vi "MTS_Main.vi"() -> ()   [LabVIEW 8.6]
panel:
  out "Pattern Y":dbl[](array[numeric])
  out "Pattern X":dbl[](array[numeric])
  out "Active pt3":path
  in  "Axis":enum32{"x-y", "x-z", "y-z"}(ring)
  in  "Save Files":bool=TRUE
  out "Intensity (a.u.)":dbl=1.0 format="%.02f"
  out "Detector2":bool
  out "Detector1":bool
  out "Excitation":bool
  in  "Measurement Time (ms)":i32=10
  in  "Open MSW":bool
  in  "New MSW":bool
  out "Workspace":path
  in  "WS File Tree":string(tree)
  out "Stop Measurement":bool
  in  "Learning loop":bool=TRUE
  in  "ShowTab":T1(tab)=enum."Auto Measurement"
  out "Video":u8[][](graph)
  in  "Find Mols":bool
  out "Image":i32[][](graph)
  in  "Save Color Image":bool
  out "AM image":T2(plugin-control)
  out "Histogram":i32[][](graph)
  out "Trace":i32[][](graph)
  out "FiFo Overrun":bool
  in  "SCANNER EMERGENCY":bool
  out "Measure. time [s]":i32
  in  "Scanner Divider":i32=2
  out "y":dbl format="%.1f nm"
  out "x":dbl format="%.1f nm"
  in  "x-Pixel":u16=100
  in  "y-Pixel":u16=100
  in  "Picture size":dbl=50.0 format="%1.1f um"
  in  "Picture size 2":dbl=50.0 format="%1.1f um"
  in  "Z-Position":dbl=50.0 caption="Z" format="%1.3f um"
  in  "Y-Position":dbl=50.0 caption="Y" format="%1.3f um"
  in  "X-Position":dbl=50.0 caption="X" format="%1.3f um"
  out "Do Measurement":T3(ring)
  in  "Point Measurement":bool
  in  "Aquire Image":bool
  in  "Settings":bool
  in  "PI E710 Port":u16(ring) items=["COM1", "COM2", "COM3", "COM4", "COM5", "COM6", "COM7", "COM8", "COM9"]
  in  "Move Stage":bool
  out "MeasRunig":bool
  in  "Stop Program":bool
  out "Global Stop":bool
  # "Workspace"
  # "Shutter:"
  # "Image Scan Settings"
  # "Point Measurement Settings"
  # "upper left corner/ Point Position"
  # "Pixelsize"
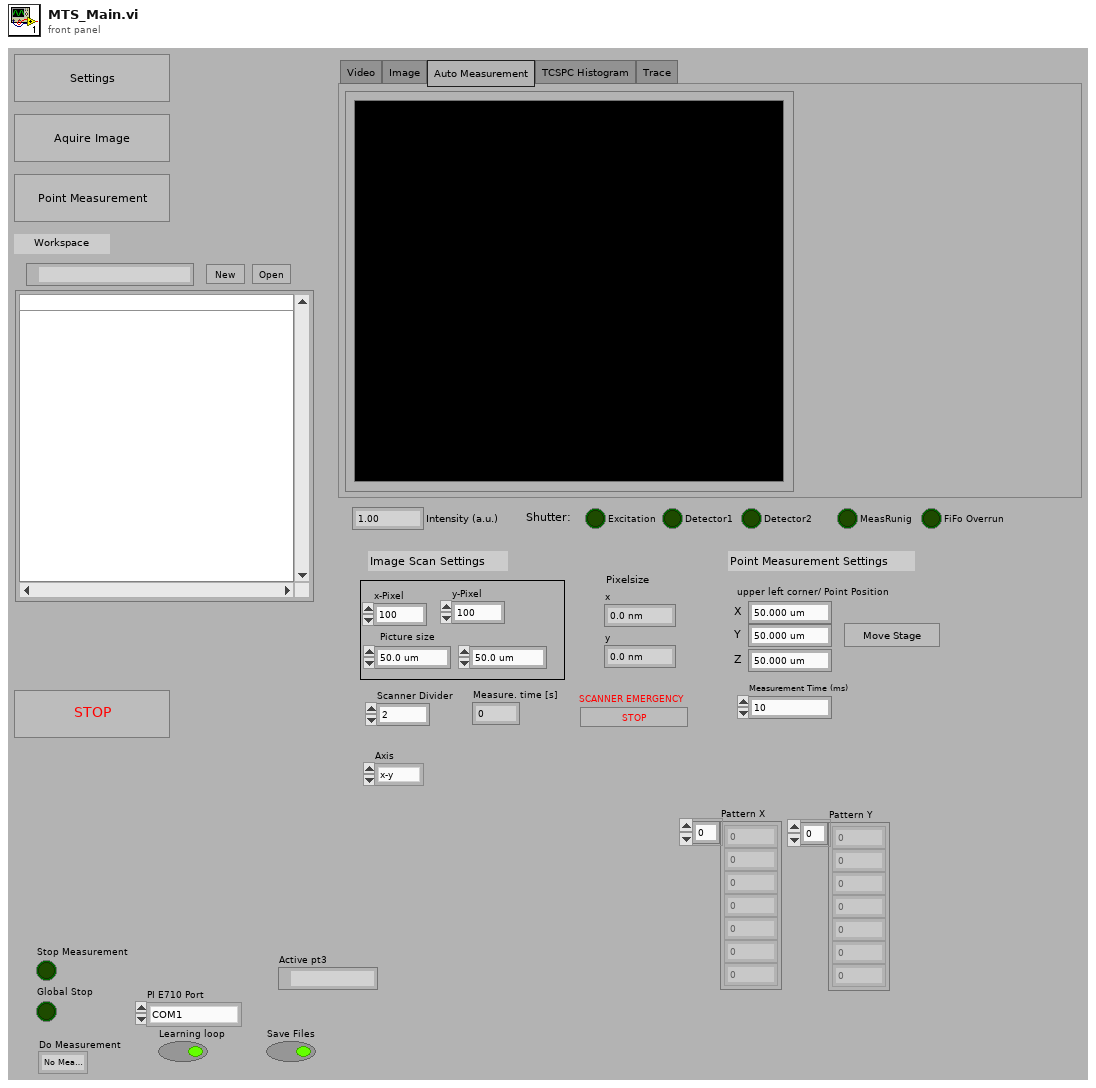
[diagram p1: front panel]
types:
  T1 = enum32{"Video", "Image", "Auto Measurement", "TCSPC Histogram", "Trace"}
  T2 = typedef "IMAQ Image.ctl" = refnum<image>
  T3 = enum16{"No Measurement", "Aquire Image", "Point Measurement", "Multi Measurement", "Save Color Image", "Find Single Mol."}
  T4 = enum16{"CAN_Baud_1M", "CAN_BAUD_500K", "CAN_BAUD_250K", "CAN_BAUD_125K", "CAN_BAUD_100K", "CAN_BAUD_50K", "CAN_BAUD_20K", "CAN_BAUD_10K", "CAN_BAUD_5K", "User"}
  T5 = enum16{"No Measurement", "Aquire Image", "Point Measurement", "Multi Measurement"}
  T6 = typedef "Image Type" = u32
  T7 = cluster{"Height":u32, "Width":u32, "Pixel Depth":u32}
  T8 = cluster{"Dev":i32, "SerNo":string, "HW_Model":string, "HW_Version":string}[]
  T9 = enum32{"Video", "Image", "TCSPC Histogram", "Trace"}
  T10 = cluster{"ID":u32, "MSG type":enum8{"STD, NO RTR", "STD,RTR", "XTD, NO RTR", "XTD, RTR"}, "LEN":u8, "DATA":u8[]}
  T11 = enum16{"No Measurement", "Aquire Image", "Point Measurement", "Multi Measurement", "Save Color Image"}
  T12 = enum16{"Get (Default)", "Set Workspace", "Append File", "Change Comment"}
  T13 = enum16{"unknown", "pt3 File", "png Image", "bmp Image"}
  T14 = cluster{"File No":i32, "File Path":path, "Parent File":i32, "File Type":enum16{"unknown", "pt3 File", "png Image", "bmp Image"}, "Measurement Type":enum16{"not a pt3 File", "Image File", "Point Measurement", "Auto Point"}, "Upper Left":cluster{"x-Position":dbl, "y-Position":dbl, "z-Position":dbl}, "Pixels":i32[], "Picture Size":dbl[], "Scan Axis":enum32{"x-y", "x-z", "y-z"}}[]
  T15 = typedef "LVPoint32TypeDef.ctl" = cluster{"Horizontal":i32, "Vertical":i32}
  T16 = cluster{"Shift":bool, "Ctrl":bool, "Alt":bool, "Cmd":bool, "Opt":bool}
  T17 = cluster{"File No":i32, "File Path":path, "Parent File":i32, "File Type":enum16{"unknown", "pt3 File", "png Image", "bmp Image"}, "Measurement Type":enum16{"not a pt3 File", "Image File", "Point Measurement", "Auto Point"}, "Upper Left":cluster{"x-Position":dbl, "y-Position":dbl, "z-Position":dbl}, "Pixels":i32[], "Picture Size":dbl[], "Scan Axis":enum32{"x-y", "x-z", "y-z"}}
  T18 = enum16{"not a pt3 File", "Image File", "Point Measurement", "Auto Point"}
  T19 = cluster{"x-Position":dbl, "y-Position":dbl, "z-Position":dbl}
  T20 = cluster{"X-Position":dbl, "Y-Position":dbl, "Z-Position":dbl}
  T21 = cluster{"Picture Size":dbl[], "Pixels":i32[], "Upper Left":cluster{"x-Position":dbl, "y-Position":dbl, "z-Position":dbl}}
  T22 = cluster{"Dev":i32, "SerNo":string, "HW_Model":string, "HW_Version":string}
  T23 = cluster{"Comment":string, "RangeNo":i32, "Offset":i32, "AcquisitionTime (ms)":i32, "HardwareSerial":i32, "SyncDivider":i32, "Resolution (ns)":sgl, "CFD Settings":cluster{"Ch0 Level":i32, "Ch0 ZeroX":i32, "Ch1 Level":i32, "Ch1 ZeroX":i32}, "InpRate0":i32, "InpRate1":i32}
  T24 = cluster{"X-Position":dbl, "Z-Position":dbl, "Y-Position":dbl}
  T25 = cluster{"Ident":string, "Format Version":string, "Creator Name":string, "Creator Version":string, "File Time":string, "Comment":string, "RangeNo":i32, "Offset":i32, "AcquisitionTime (ms)":i32, "HardwareSerial":i32, "SyncDivider":i32, "Resolution (ns)":sgl, "CFD Settings":cluster{"Ch0 Level":i32, "Ch0 ZeroX":i32, "Ch1 Level":i32, "Ch1 ZeroX":i32}, "InpRate0":i32, "InpRate1":i32}
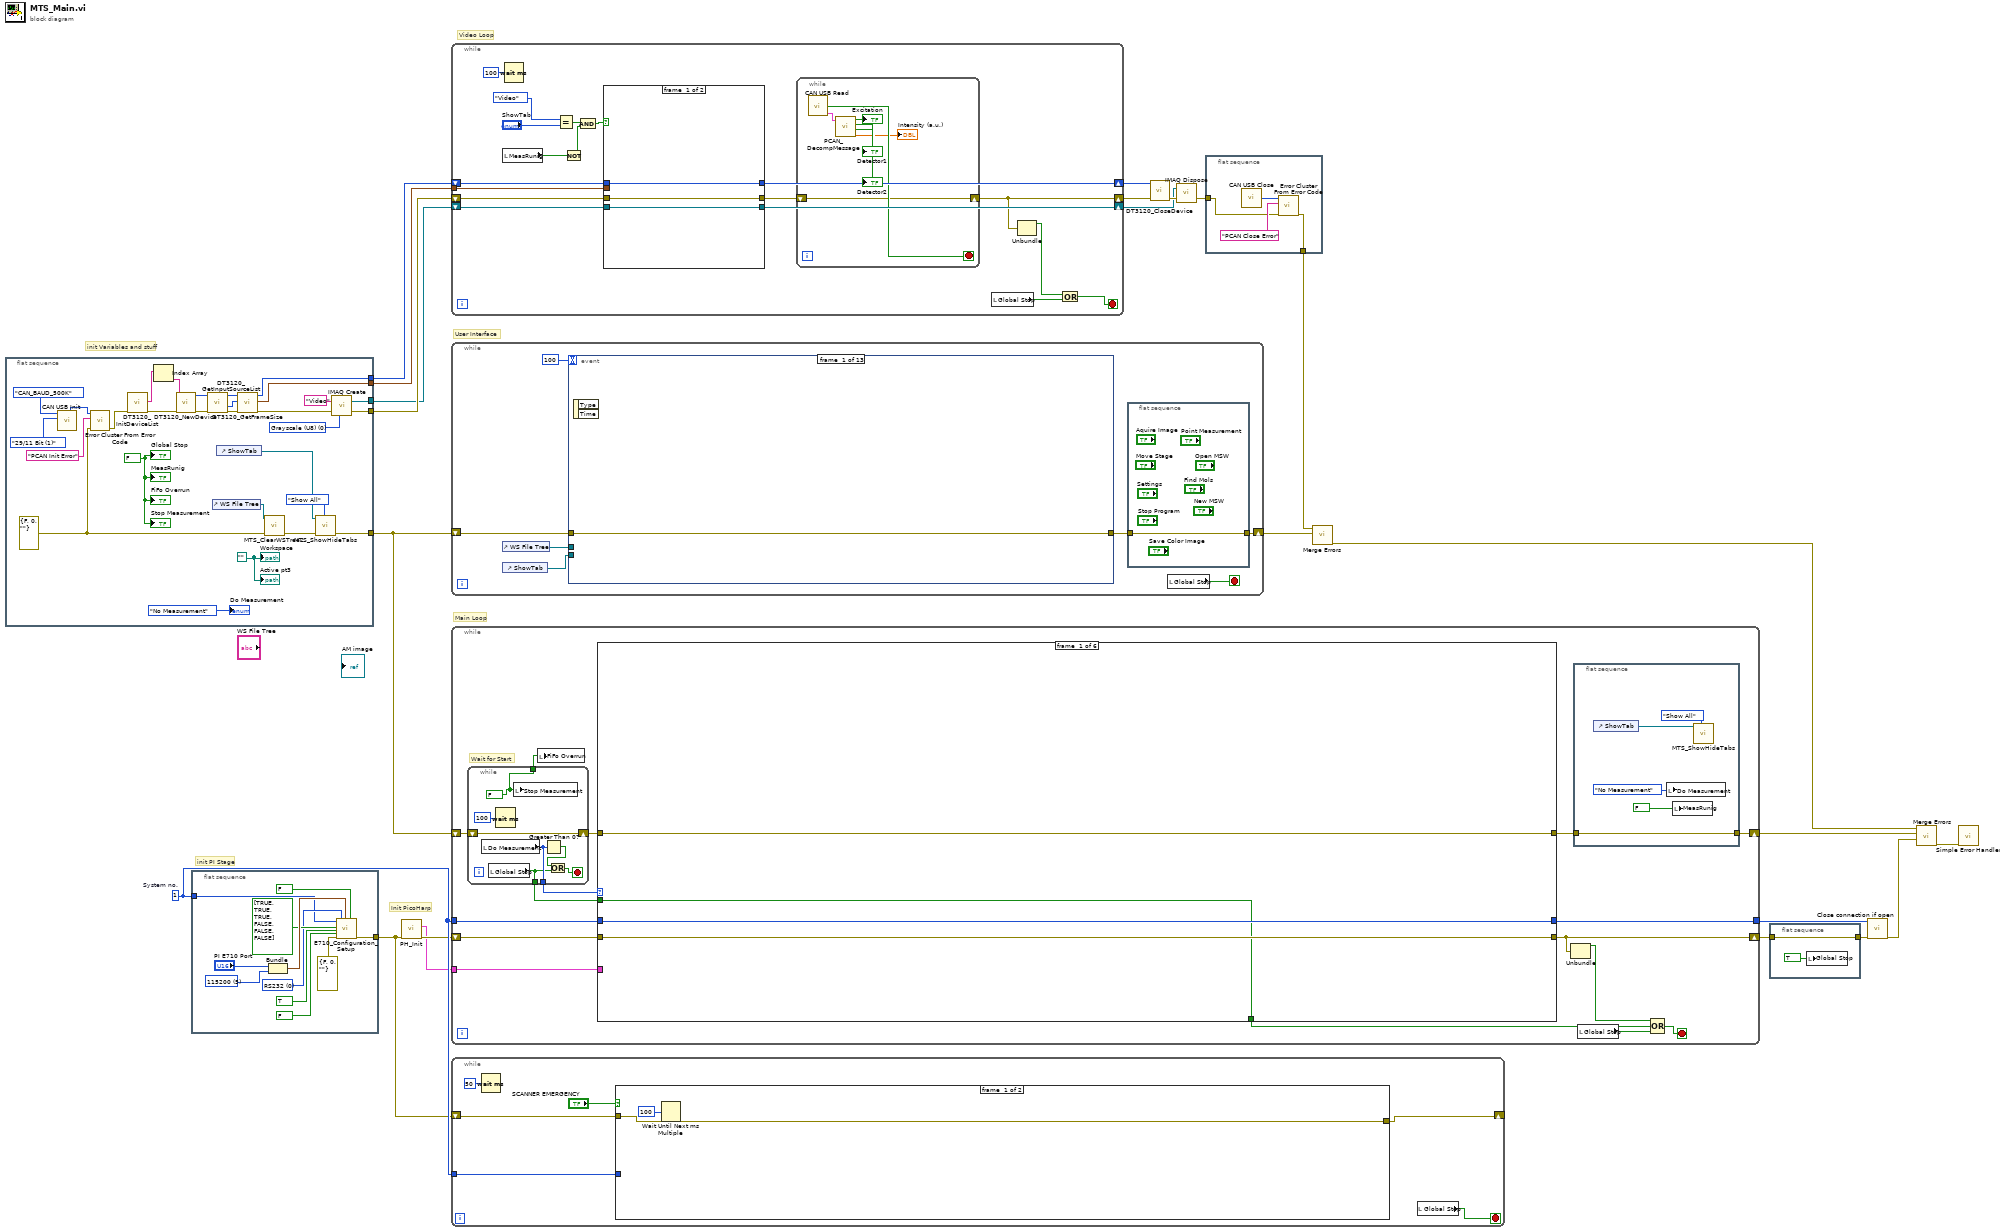
[diagram p0: block diagram]
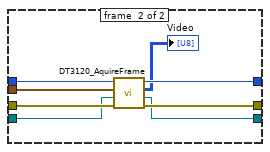
[diagram p2: hidden frame]
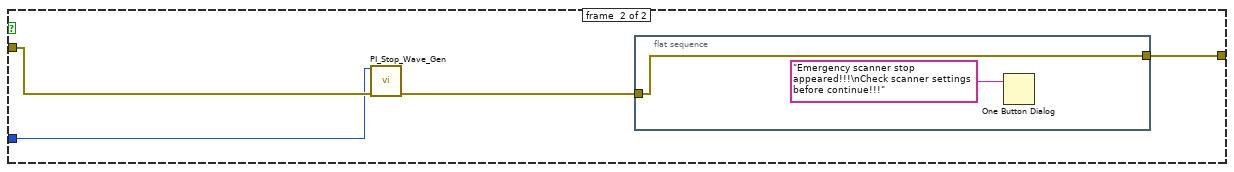
[diagram p3: hidden frame]
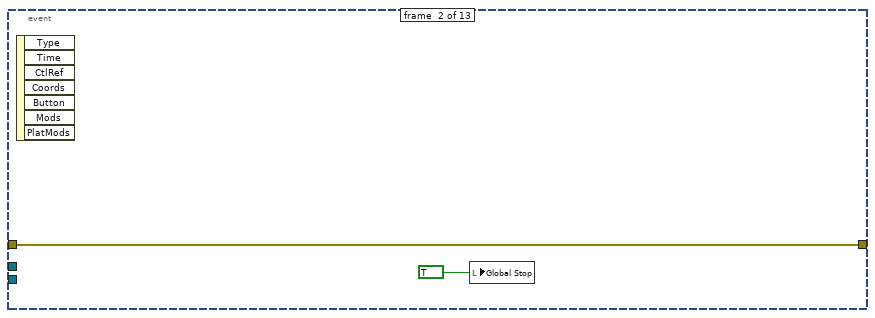
[diagram p4: hidden frame]
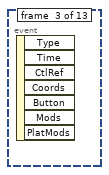
[diagram p5: hidden frame]
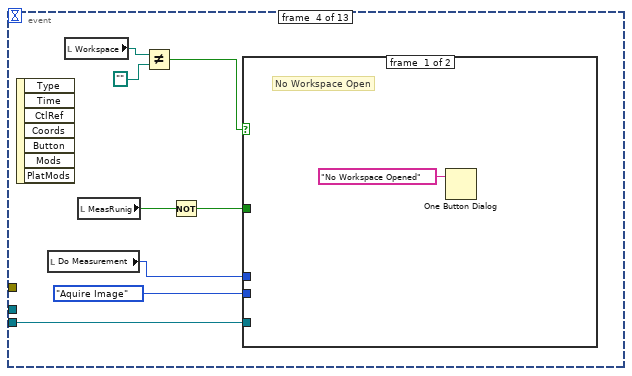
[diagram p6: hidden frame]
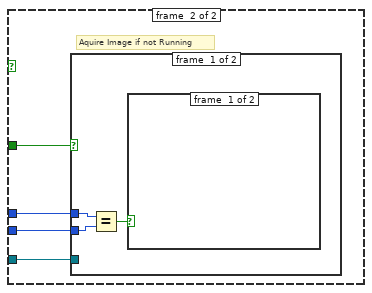
[diagram p7: hidden frame]
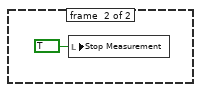
[diagram p8: hidden frame]
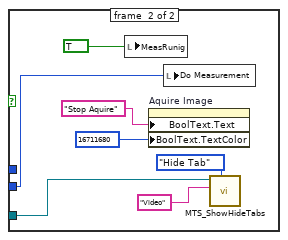
[diagram p9: hidden frame]
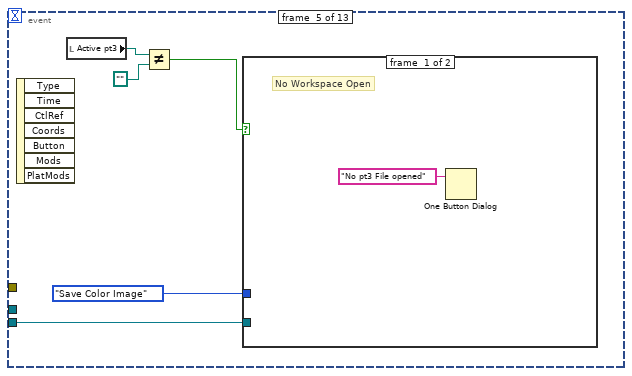
[diagram p10: hidden frame]
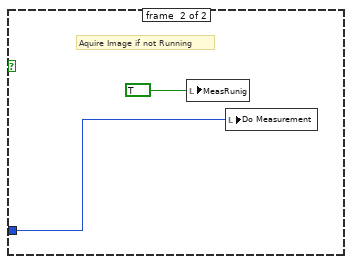
[diagram p11: hidden frame]
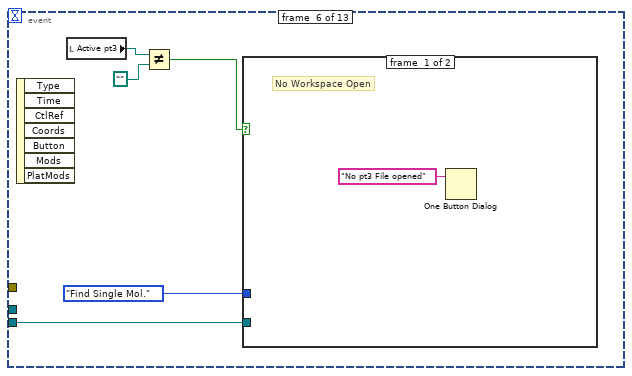
[diagram p12: hidden frame]
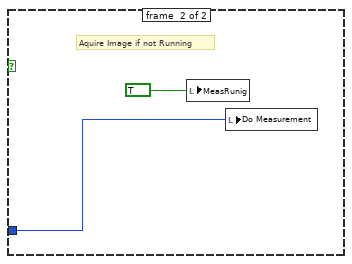
[diagram p13: hidden frame]
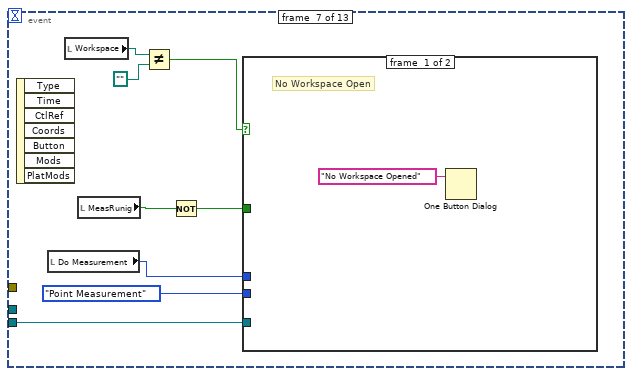
[diagram p14: hidden frame]
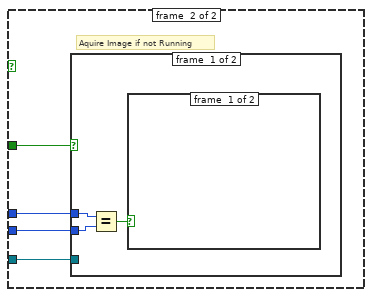
[diagram p15: hidden frame]
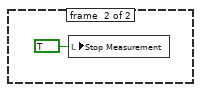
[diagram p16: hidden frame]
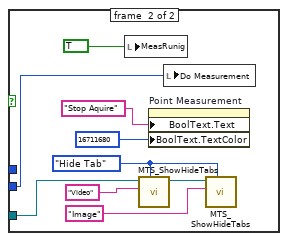
[diagram p17: hidden frame]
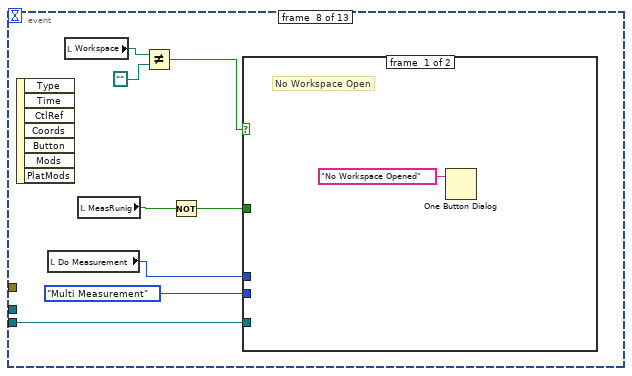
[diagram p18: hidden frame]
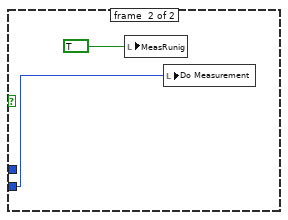
[diagram p20: hidden frame]
diagram:
  w18 = 1  # System no.
  # "Video Loop"
  # "Init PicoHarp"
  # "init Variables and stuff"
  # "User Interface"
  # "init PI Stage"
  # "Main Loop"
  n1 = flat-sequence {
    tunnel: [w33] -> w20
    tunnel: [w39] -> w12
    tunnel: [w42] -> w10
    tunnel: [w38] -> w6
    tunnel: [w37] -> w5
    frame #0 {
      w40 = T6 0 items=["Grayscale (U8)", "Grayscale (I16)", "Grayscale (SGL)", "Complex (CSG)", "RGB (U32)", "HSL (U32)", "RGB (U64)", "Grayscale (U16)"] ("Image Type")
      w24 = path ""
      w27 = errorcluster {"status"=FALSE, "code"=0, "source"=""} ("error in")
      w51 = FALSE ("Global Stop")
      n2 = call "CAN USB Init.vi"("CAN Msg Type"=enum16{"11 Bit (0)", "29/11 Bit (1)"}."29/11 Bit (1)", "BTR0BTR1"=T4."CAN_BAUD_500K") -> ("Error Number"=w28:u32)  [unwired: 7 in, 2 out]
      n3 = call <vilib>:"Error Cluster From Error Code.vi"("error in (no error)"=w27, "error message (\"\")"="PCAN Init Error" ("error message (\"\")"), "error code (0)"=w28) -> ("error out"=w26:errorcluster)  [unwired: 6 in]
      n4 = call "DT3120_InitDeviceList.vi"("error in (no error)"=w26) -> ("error out"=w49:errorcluster, "Alias List"=w50:string[])  [unwired: 9 out]
      n5 = Index Array(array=w50) -> (element=w48:string)  [unwired: 1 in]
      n6 = call "DT3120_NewDevice.vi"("error in (no error)"=w49, "Alias"=w48) -> ("error out"=w44:errorcluster, "DevId"=w43:i32)  [unwired: 8 out]
      n7 = call "DT3120_GetInputSourceList.vi"("error in (no error)"=w44, "DevId"=w43) -> ("error out"=w47:errorcluster, "Active Source"=w46:u16, "DevId (dup)"=w45:i32)  [unwired: 7 out]
      n8 = control-ref of="WS File Tree"() -> (w35:refnum<vi>)
      n9 = control-ref of="ShowTab"() -> (w32:refnum<vi>)
      n10 = call "DT3120_GetFrameSize.vi"("error in (no error)"=w47, "Source"=w46, "DevId"=w45) -> ("error out"=w41:errorcluster, "Frame Size"=w38:T7, "DevId (dup)"=w42:i32)  [unwired: 6 in]
      n11 = call "MTS_ClearWSTree2.vi"("error in"=w27, "Tree Refnum"=w35) -> ("error out"=w34:errorcluster)  [unwired: 8 in, 1 out]
      n12 = call "MTS_ShowHideTabs.vi"("Action"=enum16{"Show All", "Hide Tab", "Show Tab"}."Show All", "error in (no error)"=w34, "ShowTab"=w32) -> ("error out"=w33:errorcluster)  [unwired: 7 in, 1 out]
      n13 = call "IMAQ Create"("Image Name"="Video", "Image Type"=w40, "error in (no error)"=w41) -> ("New Image"=w37:T2, "error out"=w39:errorcluster)  [unwired: 2 in]
      "Global Stop" <- w51
      "MeasRunig" <- w51
      "Do Measurement" <- T5."No Measurement" ("Do Measurement")
      "FiFo Overrun" <- w51
      "Stop Measurement" <- w51
      "Workspace" <- w24
      "Active pt3" <- w24
    }
  }
  n14 = flat-sequence {
    tunnel: [w55] -> w17
    tunnel: w18 -> [w54]
    frame #0 {
      w62 = u16 5 items=["9600", "14400", "19200", "38400", "57600", "115200"] ("Baudrate")
      w57 = u16 0 items=["RS232", "GPIB"] ("Interface")
      n15 = Bundle("PI E710 Port"="PI E710 Port", "Baudrate"=w62) -> (w63:cluster{"PI E710 Port":u16, "Baudrate":u16})  [unwired: 1 out]
      n16 = call <userlib>:"E710_Configuration_Setup.vi"("System no."=w54, "Are stages connected?"=bool[] [TRUE, TRUE, TRUE, FALSE, FALSE, FALSE], "Change servo \nstatus to ON?"=TRUE ("Change servo \nstatus to ON?"), "Perform autozero?"=FALSE ("All axes?"), "error in"=errorcluster {"status"=FALSE, "code"=0, "source"=""}, "Interface"=w57, "RS232 settings"=w63, "Move to middle?"=FALSE) -> ("error out"=w55:errorcluster)  [unwired: 4 in, 7 out]
    }
  }
  n17 = call "PH_Init.vi"("error in (no error)"=w17) -> ("Device List"=w15:T8, "error out"=w16:errorcluster)  [unwired: 12 in, 1 out]
  n18 = while {
    shift-right: [w64] -> w11
    shift-left: w12 -> [w78]
    shift-right: [w71] -> w9
    shift-left: w10 -> [w72]
    tunnel: w6 -> [w73]
    shift-right: [w70] -> w3
    shift-left: w5 -> [w74]
    stop <- w77 stop-if-true
    n19 = local read "MeasRunig"() -> (w69:bool)
    n20 = Wait (ms)(milliseconds to wait=u32 100) -> ()  [unwired: 1 out]
    n21 = Equal?(x=T9."Video" ("ShowTab"), y="ShowTab") -> (x = y?=w68:bool)
    n22 = Not(x=w69) -> (.not. x?=w66:bool)
    n23 = And(x=w68, y=w66) -> (x .and. y?=w67:bool)
    n24 = case shown="True" w67 {
      tunnel: w78 -> [w91 w99]
      tunnel: [w91 w98] -> w65
      tunnel: w74 -> [w89 w97]
      tunnel: w73 -> [_ w96]
      tunnel: w72 -> [w90 w95]
      tunnel: [w90 w94] -> w71
      tunnel: [w89 w93] -> w70
      frame #0 {
      }
      frame #1 {
        n25 = call "DT3120_AquireFrame.vi"("error in (no error)"=w99, "Image"=w97, "Frame Size"=w96, "DevId"=w95) -> ("error out"=w98:errorcluster, "Image Out"=w93:T2, "Frame"=→"Video":u8[][], "DevId (dup)"=w94:i32)  [unwired: 4 in]
      }
    }
    n26 = while {
      shift-right: [w83] -> w64
      shift-left: w65 -> [w83]
      stop <- w88 stop-if-true
      n27 = call "CAN USB Read.vi"() -> ("RcvQueueEmpty"=w88:bool, "CAN_Message out"=w87:T10)  [unwired: 1 in, 1 out]
      n28 = call "PCAN_DecompMessage.vi"("CAN_Message out"=w87) -> ("Intensity (a.u.)"=→"Intensity (a.u.)":dbl, "Detector2 Shutter Open?"=→"Detector2":bool, "Detector1 Shutter Open?"=→"Detector1":bool, "Excitation Shutter Open?"=→"Excitation":bool)  [unwired: 7 in]
    }
    n29 = local read "Global Stop"() -> (w76:bool)
    n30 = Unbundle(w64) -> ("status"=w75:bool)  [unwired: 2 out]
    n31 = Compound Arithmetic op=OR(w75, w76) -> (w77:bool)
  }
  n32 = while {
    shift-right: [w104] -> w8
    shift-left: w20 -> [w105]
    stop <- w102 stop-if-true
    n33 = control-ref of="WS File Tree"() -> (w101:refnum<vi>)
    n34 = control-ref of="ShowTab"() -> (w100:refnum<vi>)
    n35 = event shown="[3] \"Aquire Image\": Mouse Up" {
      selector: _ -> [_ _ _ _ _ _ _ _ _ _ _ _ _]
      dyn-events: _ -> [_ _ _ _ _ _ _ _ _ _ _ _ _]
      timeout: 100 -> [_ _ _ _ _ _ _ _ _ _ _ _ _]
      tunnel: w105 -> [w108 w110 _ _ _ _ _ _ w194 w230 _ w282 _]
      tunnel: [w108 w110 _ _ _ _ _ _ w192 w227 _ w281 _] -> w103
      tunnel: w101 -> [_ _ _ _ _ _ _ _ w196 w231 _ _ _]
      tunnel: w100 -> [_ _ _ w111 w135 w143 w151 w177 _ _ _ _ _]
      event #0 {
        n36 = event-data() -> ()  [unwired: 1 in, 2 out]
      }
      event #1 {
        n37 = event-data() -> ()  [unwired: 1 in, 7 out]
        n38 = local write "Global Stop"(TRUE ("Global Stop")) -> ()
      }
      event #2 {
        n39 = event-data() -> ()  [unwired: 1 in, 7 out]
      }
      event #3 {
        n40 = event-data() -> ()  [unwired: 1 in, 7 out]
        n41 = local read "Do Measurement"() -> (w115:T3)
        n42 = local read "Workspace"() -> (w114:path)
        n43 = local read "MeasRunig"() -> (w118:bool)
        n44 = Not Equal?(x=w114, y=path "") -> (x != y?=w112:bool)
        n45 = Not(x=w118) -> (.not. x?=w117:bool)
        n46 = case shown="True" w112 {
          tunnel: w117 -> [_ w123]
          tunnel: T11."Aquire Image" ("Do Measurement") -> [_ w122]
          tunnel: w115 -> [_ w121]
          tunnel: w111 -> [_ w120]
          frame #0 {
            # "No Workspace Open"
            n47 = One Button Dialog(message="No Workspace Opened") -> ()  [unwired: 1 in, 1 out]
          }
          frame #1 {
            # "Aquire Image if not Running"
            n48 = case shown="True" w123 {
              tunnel: w122 -> [w125 w132]
              tunnel: w121 -> [w126 _]
              tunnel: w120 -> [_ w128]
              frame #0 {
                n49 = Equal?(x=w126, y=w125) -> (x = y?=w124:bool)
                n50 = case shown="True" w124 {
                  frame #0 {
                  }
                  frame #1 {
                    n51 = local write "Stop Measurement"(TRUE ("Stop Measurement")) -> ()
                  }
                }
              }
              frame #1 {
                n52 = local write "MeasRunig"(TRUE ("Measurement Running")) -> ()
                n53 = property on="Aquire Image" class="Bool"("BoolText.Text"="Stop Aquire" ("Caption.Text"), "BoolText.TextColor"=u32 16711680 ("Boolean Text.Colors:FG Color")) -> ()  [unwired: 2 in, 2 out]
                n54 = local write "Do Measurement"(w132) -> ()
                n55 = call "MTS_ShowHideTabs.vi"("Action"=enum16{"Show All", "Hide Tab", "Show Tab"}."Hide Tab", "Tab Caption"="Video", "ShowTab"=w128) -> ()  [unwired: 7 in, 2 out]
              }
            }
          }
        }
      }
      event #4 {
        n56 = event-data() -> ()  [unwired: 1 in, 7 out]
        n57 = local read "Active pt3"() -> (w138:path)
        n58 = Not Equal?(x=w138, y=path "") -> (x != y?=w136:bool)
        n59 = case shown="True" w136 {
          tunnel: T3."Save Color Image" ("Do Measurement") -> [_ w142]
          tunnel: w135 -> [_ _]
          frame #0 {
            # "No Workspace Open"
            n60 = One Button Dialog(message="No pt3 File opened") -> ()  [unwired: 1 in, 1 out]
          }
          frame #1 {
            # "Aquire Image if not Running"
            n61 = local write "MeasRunig"(TRUE ("Measurement Running")) -> ()
            n62 = local write "Do Measurement"(w142) -> ()
          }
        }
      }
      event #5 {
        n63 = event-data() -> ()  [unwired: 1 in, 7 out]
        n64 = local read "Active pt3"() -> (w146:path)
        n65 = Not Equal?(x=w146, y=path "") -> (x != y?=w144:bool)
        n66 = case shown="True" w144 {
          tunnel: T3."Find Single Mol." ("Do Measurement") -> [_ w150]
          tunnel: w143 -> [_ _]
          frame #0 {
            # "No Workspace Open"
            n67 = One Button Dialog(message="No pt3 File opened") -> ()  [unwired: 1 in, 1 out]
          }
          frame #1 {
            # "Aquire Image if not Running"
            n68 = local write "MeasRunig"(TRUE ("Measurement Running")) -> ()
            n69 = local write "Do Measurement"(w150) -> ()
          }
        }
      }
      event #6 {
        n70 = event-data() -> ()  [unwired: 1 in, 7 out]
        n71 = local read "Do Measurement"() -> (w155:T3)
        n72 = local read "Workspace"() -> (w154:path)
        n73 = local read "MeasRunig"() -> (w158:bool)
        n74 = Not Equal?(x=w154, y=path "") -> (x != y?=w152:bool)
        n75 = Not(x=w158) -> (.not. x?=w157:bool)
        n76 = case shown="True" w152 {
          tunnel: w157 -> [_ w163]
          tunnel: T11."Point Measurement" ("Do Measurement") -> [_ w162]
          tunnel: w155 -> [_ w161]
          tunnel: w151 -> [_ w160]
          frame #0 {
            # "No Workspace Open"
            n77 = One Button Dialog(message="No Workspace Opened") -> ()  [unwired: 1 in, 1 out]
          }
          frame #1 {
            # "Aquire Image if not Running"
            n78 = case shown="True" w163 {
              tunnel: w162 -> [w165 w174]
              tunnel: w161 -> [w166 _]
              tunnel: w160 -> [_ w171]
              frame #0 {
                n79 = Equal?(x=w166, y=w165) -> (x = y?=w164:bool)
                n80 = case shown="True" w164 {
                  frame #0 {
                  }
                  frame #1 {
                    n81 = local write "Stop Measurement"(TRUE ("Stop Measurement")) -> ()
                  }
                }
              }
              frame #1 {
                w168 = enum16{"Show All", "Hide Tab", "Show Tab"}."Hide Tab" ("Action")
                n82 = local write "MeasRunig"(TRUE ("Measurement Running")) -> ()
                n83 = call "MTS_ShowHideTabs.vi"("Action"=w168, "Tab Caption"="Video", "ShowTab"=w171) -> ("ShowTab (dup)"=w170:refnum<vi>)  [unwired: 7 in, 1 out]
                n84 = property on="Point Measurement" class="Bool"("BoolText.Text"="Stop Aquire" ("Caption.Text"), "BoolText.TextColor"=u32 16711680 ("Boolean Text.Colors:FG Color")) -> ()  [unwired: 2 in, 2 out]
                n85 = local write "Do Measurement"(w174) -> ()
                n86 = call "MTS_ShowHideTabs.vi"("Action"=w168, "Tab Caption"="Image", "ShowTab"=w170) -> ()  [unwired: 7 in, 2 out]
              }
            }
          }
        }
      }
      event #7 {
        n87 = event-data() -> ()  [unwired: 1 in, 7 out]
        n88 = local read "Do Measurement"() -> (w181:T3)
        n89 = local read "Workspace"() -> (w180:path)
        n90 = local read "MeasRunig"() -> (w184:bool)
        n91 = Not Equal?(x=w180, y=path "") -> (x != y?=w178:bool)
        n92 = Not(x=w184) -> (.not. x?=w183:bool)
        n93 = case shown="True" w178 {
          tunnel: w183 -> [_ w189]
          tunnel: T11."Multi Measurement" ("Do Measurement") -> [_ w188]
          tunnel: w181 -> [_ w187]
          tunnel: w177 -> [_ w186]
          frame #0 {
            # "No Workspace Open"
            n94 = One Button Dialog(message="No Workspace Opened") -> ()  [unwired: 1 in, 1 out]
          }
          frame #1 {
            # "Aquire Image if not Running"
            n95 = case shown="True" w189 {
              tunnel: w188 -> [_ w190]
              tunnel: w187 -> [_ _]
              tunnel: w186 -> [_ _]
              frame #0 {
              }
              frame #1 {
                n96 = local write "MeasRunig"(TRUE ("Measurement Running")) -> ()
                n97 = local write "Do Measurement"(w190) -> ()
              }
            }
          }
        }
      }
      event #8 {
        # "Default Name"
        n98 = event-data() -> ()  [unwired: 1 in, 7 out]
        n99 = flat-sequence {
          tunnel: [w212] -> w195
          tunnel: w194 -> [w212]
          frame #0 {
            n100 = local write "MeasRunig"(TRUE ("MeasRunig")) -> ()
          }
        }
        n101 = Get Date/Time In Seconds() -> (seconds since 1Jan1904=w209:timestamp)
        n102 = Format Date/Time String(time format string (%c)="%Y-%m-%d", seconds (now)=w209) -> (date/time string=w207:string)  [unwired: 1 out]
        n103 = Concatenate Strings(w207, ".msw" ("string")) -> (w205:string)
        n104 = call "File Dialog"("start path"=path "E:/", "prompt"="Create New Workspace", "button label"="Create", "default name"=w205, "error in"=w195, "pattern (all files)"="*.msw", "pattern label"="MT Scan Workspace") -> ("selected path"=w199:path, "cancelled"=w200:bool, "error out"=w198:errorcluster)  [unwired: 5 in, 1 out]
        n105 = case shown="False" w200 {
          tunnel: w199 -> [w218 _]
          tunnel: w198 -> [w224 w226]
          tunnel: [w216 w225] -> w193
          tunnel: w196 -> [w214 _]
          frame #0 {
            # "Create Empty Workspace"
            n106 = local write "Workspace"(w218) -> ()
            n107 = call "MTS_CreateWriteMSW.vi"("Rewrite"=TRUE, "error in (no error)"=w224, "Workspace Path"=w218) -> ("error out"=w217:errorcluster, "Created"=w221:string, "Comment (dup)"=w220:string, "Files in Workspace (dup)"=w219:T14)  [unwired: 5 in]
            n108 = call "MTS_Workspace.vi"("Workspace"=w218, "Operation"=T12."Set Workspace", "Created in"=w221, "New Comment"=w220, "Files in Workspace in"=w219) -> ("Files in Workspace"=w215:T14)  [unwired: 3 in, 3 out]
            n109 = call "MTS_BuildWSTree.vi"("error in"=w217, "Files in Workspace"=w215, "Tree Refnum"=w214) -> ("error out"=w216:errorcluster)  [unwired: 7 in, 1 out]
          }
          frame #1 {
            n110 = call <vilib>:"Clear Errors.vi"("error in (no error)"=w226) -> ("error out"=w225:errorcluster)  [unwired: 6 in]
          }
        }
        n111 = flat-sequence {
          tunnel: w193 -> [w210]
          tunnel: [w210] -> w192
          frame #0 {
            n112 = local write "MeasRunig"(FALSE ("MeasRunig")) -> ()
          }
        }
      }
      event #9 {
        n113 = event-data() -> ()  [unwired: 1 in, 7 out]
        n114 = flat-sequence {
          tunnel: w230 -> [w242]
          tunnel: [w242] -> w229
          frame #0 {
            n115 = local write "MeasRunig"(TRUE ("MeasRunig")) -> ()
          }
        }
        n116 = call "File Dialog2"("start path"=path "E:/", "prompt"="Create New Workspace", "button label"="Open", "error in"=w229, "pattern (all files)"="*.msw", "pattern label"="MT Scan Workspace") -> ("selected path"=w234:path, "cancelled"=w235:bool, "error out"=w233:errorcluster)  [unwired: 6 in, 1 out]
        n117 = case shown="False" w235 {
          tunnel: w234 -> [w248 _]
          tunnel: w233 -> [w253 w255]
          tunnel: [w246 w254] -> w228
          tunnel: w231 -> [w244 _]
          frame #0 {
            # "Open Workspace"
            n118 = local write "Workspace"(w248) -> ()
            n119 = call "MTS_ReadMSW.vi"("error in (no error)"=w253, "Workspace Path"=w248) -> ("error out"=w247:errorcluster, "Created"=w251:string, "Comment"=w250:string, "Files in Workspace"=w249:T14)  [unwired: 6 in]
            n120 = call "MTS_Workspace.vi"("Workspace"=w248, "Operation"=T12."Set Workspace", "Created in"=w251, "New Comment"=w250, "Files in Workspace in"=w249) -> ("Files in Workspace"=w245:T14)  [unwired: 3 in, 3 out]
            n121 = call "MTS_BuildWSTree.vi"("error in"=w247, "Files in Workspace"=w245, "Tree Refnum"=w244) -> ("error out"=w246:errorcluster)  [unwired: 7 in, 1 out]
          }
          frame #1 {
            n122 = call <vilib>:"Clear Errors.vi"("error in (no error)"=w255) -> ("error out"=w254:errorcluster)  [unwired: 6 in]
          }
        }
        n123 = flat-sequence {
          tunnel: w228 -> [w240]
          tunnel: [w240] -> w227
          frame #0 {
            n124 = local write "MeasRunig"(FALSE ("MeasRunig")) -> ()
          }
        }
      }
      event #10 {
        w258 = 100.0 ("y")
        n125 = event-data() -> ("Coords"=w270:T15, "PlatMods"=w271:T16)  [unwired: 1 in, 5 out]
        n126 = local read "Axis"() -> (w266:enum32{"x-y", "x-z", "y-z"})
        n127 = invoke on="Image" class="IntGraph (strict)" method="Map Coords To XY"("Coords"=w270) -> ("Map Coords To XY"=w267:bool, "XY"=w265:cluster{"X":dbl, "Y":dbl})  [unwired: 6 in, 5 out]
        n128 = Unbundle By Name(w271) -> ("Ctrl"=w268:bool)
        n129 = And(x=w267, y=w268) -> (x .and. y?=w269:bool)
        n130 = Unbundle(w265) -> ("X"=w264:dbl, "Y"=w261:dbl)
        n131 = Multiply(x=w264, y=w258) -> (x*y=w263:dbl)
        n132 = Multiply(x=w261, y=w258) -> (x*y=w260:dbl)
        n133 = Round To Nearest(number=w263) -> (nearest integer value=w262:dbl)
        n134 = Round To Nearest(number=w260) -> (nearest integer value=w259:dbl)
        n135 = Divide(x=w262, y=w258) -> (x/y=w257:dbl)
        n136 = Divide(x=w259, y=w258) -> (x/y=w256:dbl)
        n137 = case shown="True" w269 {
          tunnel: w266 -> [_ w274]
          tunnel: w257 -> [_ w273]
          tunnel: w256 -> [_ w272]
          frame #0 {
          }
          frame #1 {
            n138 = case shown="\"x-y\", Default" w274 {
              tunnel: w273 -> [w276 w278 w280]
              tunnel: w272 -> [w275 w277 w279]
              frame #0 {
                n139 = local write "X-Position"(w276) -> ()
                n140 = local write "Y-Position"(w275) -> ()
              }
              frame #1 {
                n141 = local write "X-Position"(w278) -> ()
                n142 = local write "Z-Position"(w277) -> ()
              }
              frame #2 {
                n143 = local write "Y-Position"(w280) -> ()
                n144 = local write "Z-Position"(w279) -> ()
              }
            }
          }
        }
      }
      event #11 {
        n145 = event-data() -> ("NewVal"=w286:string)  [unwired: 1 in, 4 out]
        n146 = local read "Workspace"() -> (w283:path)
        n147 = Not Equal?(x=w283, y=path "") -> (x != y?=w284:bool)
        n148 = case shown="True" w284 {
          tunnel: w286 -> [_ w297]
          tunnel: w283 -> [_ w296]
          tunnel: w282 -> [w287 w295]
          tunnel: [w287 w294] -> w281
          frame #0 {
          }
          frame #1 {
            n149 = call "MTS_GetFileFromWS.vi"("Tree Label"=w297) -> ("File Header"=w293:T17, "File Found"=w292:bool)  [unwired: 9 in]
            n150 = Unbundle By Name(w293) -> ("File Type"=w291:T13)
            n151 = Equal?(x=w291, y=T13."pt3 File" ("File Type")) -> (x = y?=w289:bool)
            n152 = And(x=w292, y=w289) -> (x .and. y?=w288:bool)
            n153 = case shown="True" w288 {
              tunnel: w293 -> [_ w317]
              tunnel: w296 -> [_ w323]
              tunnel: w295 -> [w298 w318]
              tunnel: [w298 w305] -> w294
              frame #0 {
              }
              frame #1 {
                # "Image Intensity Array"
                n154 = Unbundle By Name(w317) -> ("Measurement Type"=w304:T18, "Pixels"=w302:i32[], "Picture Size"=w301:dbl[], "Upper Left"=w300:T19, "Scan Axis"=w299:enum32{"x-y", "x-z", "y-z"})
                n155 = Unbundle By Name(w317) -> ("File Path"=w322:path)
                n156 = Strip Path(path=w323) -> (stripped path=w321:path)  [unwired: 1 out]
                n157 = Strip Path(path=w322) -> (name=w320:string)  [unwired: 1 out]
                n158 = control-ref of="Image"() -> (w303:refnum<vi>)
                n159 = Build Path(base path=w321, name or relative path=w320) -> (appended path=w319:path)
                n160 = Index Array(array=w302, index #2=1 ("index")) -> (element #1=w314:i32, element #2=w313:i32)  [unwired: 1 in]
                n161 = call "PT3_Open.vi"("error in"=w318, "File Path"=w319) -> ("error out"=w312:errorcluster, "refnum out"=w311:refnum<file>)  [unwired: 4 in, 4 out]
                n162 = local write "Active pt3"(w319) -> ()
                n163 = Initialize Array(0 ("element"), w314, w313) -> (w310:i32[][])
                n164 = case shown="\"Image File\"" w304 {
                  tunnel: w312 -> [w330 w362]
                  tunnel: w311 -> [w337 w361]
                  tunnel: w310 -> [w336 w360]
                  tunnel: [w334 w359] -> w309
                  tunnel: [w333 w358] -> w308
                  tunnel: [w332 w357] -> w307
                  tunnel: [w331 w356] -> w306
                  tunnel: w303 -> [w328 _]
                  tunnel: w302 -> [w327 _]
                  tunnel: w301 -> [w326 _]
                  tunnel: w300 -> [w325 _]
                  tunnel: w299 -> [w324 _]
                  frame #0 {
                    n165 = call "MTS_SetGraphScales.vi"("Pixels"=w327, "Axis"=w324, "Picture Size"=w326, "error in (no error)"=w330, "Upper Left"=w325, "Image"=w328) -> ("error out"=w329:errorcluster)  [unwired: 5 in]
                    n166 = while {
                      tunnel: w337 -> [w352]
                      shift-right: [FALSE ("Start From Top")] -> _
                      shift-left: TRUE ("Start From Top") -> [w346]
                      shift-right: [w345] -> w331
                      shift-left: w329 -> [w341]
                      tunnel: [w344] -> w332
                      tunnel: [w343] -> w334
                      tunnel: [w342] -> w335
                      tunnel: w336 -> [w340]
                      tunnel: [w339] -> w333
                      stop <- w349 stop-if-true
                      n167 = call "PT3_Read.vi"("Start From Top"=w346, "error in"=w341, "Data count"=10000, "refnum in"=w352) -> ("error out"=w345:errorcluster, "Data out"=w348:u32[], "refnum out"=w344:refnum<file>, "EOF?"=w349:bool)  [unwired: 4 in]
                      n168 = Array Size(array=w348) -> (size(s)=w347:i32)
                      n169 = call "MTS_ToImageOffline.vi"("Data In"=w348, "Reset"=w346, "Image Array In"=w340, "Data Count"=w347) -> ("Image Array Out"=w342:i32[][], "Histograms"=w343:i32[][], "Traces"=w339:i32[][])  [unwired: 2 in, 7 out]
                    }
                    n170 = local write "Image"(w335) -> ()
                  }
                  frame #1 {
                    w363 = TRUE ("Start From Top")
                    n171 = call "PT3_Read.vi"("Start From Top"=w363, "error in"=w362, "Data count"=10000, "refnum in"=w361) -> ("error out"=w356:errorcluster, "Data out"=w354:u32[], "refnum out"=w357:refnum<file>)  [unwired: 4 in, 1 out]
                    n172 = Array Size(array=w354) -> (size(s)=w353:i32)
                    n173 = call "MTS_ToImageOffline.vi"("Data In"=w354, "Reset"=w363, "Image Array In"=w360, "Data Count"=w353) -> ("Histograms"=w359:i32[][], "Traces"=w358:i32[][])  [unwired: 2 in, 8 out]
                  }
                }
                n174 = local write "Histogram"(w309) -> ()
                n175 = local write "Trace"(w308) -> ()
                n176 = Close File(refnum=w307, error in=w306) -> (error out=w305:errorcluster)  [unwired: 1 out]
              }
            }
          }
        }
      }
      event #12 {
        w366 = 1000.0 ("y")
        n177 = event-data() -> ()  [unwired: 1 in, 5 out]
        n178 = local read "Picture size 2"() -> (w368:dbl)
        n179 = local read "Picture size"() -> (w372:dbl)
        n180 = local read "x-Pixel"() -> (w371:u16)
        n181 = local read "y-Pixel"() -> (w367:u16)
        n182 = Divide(x=w372, y=w371) -> (x/y=w370:dbl)
        n183 = Divide(x=w368, y=w367) -> (x/y=w369:dbl)
        n184 = Multiply(x=w370, y=w366) -> (x*y=→"x":dbl)
        n185 = Multiply(x=w369, y=w366) -> (x*y=→"y":dbl)
      }
    }
    n186 = flat-sequence {
      tunnel: [w107] -> w104
      tunnel: w103 -> [w107]
      frame #0 {
      }
    }
    n187 = local read "Global Stop"() -> (w102:bool)
  }
  n188 = while {
    shift-right: [w375] -> w14
    shift-left: w16 -> [w387]
    tunnel: w18 -> [w386]
    tunnel: [w385] -> w23
    shift-right: [w377] -> w19
    shift-left: w20 -> [w388]
    tunnel: w15 -> [w376]
    stop <- w383 stop-if-true
    # "Wait for Start"
    n189 = while {
      shift-right: [w852] -> w379
      shift-left: w388 -> [w852]
      tunnel: [w849] -> w381
      tunnel: [w848] -> w380
      tunnel: [w847] -> w373
      stop <- w853 stop-if-true
      w847 = FALSE ("FiFo Overrun")
      n190 = local read "Do Measurement"() -> (w849:T3)
      n191 = local read "Global Stop"() -> (w848:bool)
      n192 = Wait (ms)(milliseconds to wait=u32 100) -> ()  [unwired: 1 out]
      n193 = local write "Stop Measurement"(w847) -> ()
      n194 = Greater Than 0?(x=w849) -> (x > 0?=w851:bool)
      n195 = Or(x=w851, y=w848) -> (x .or. y?=w853:bool)
    }
    n196 = local write "FiFo Overrun"(w373) -> ()
    n197 = case shown="\"Point Measurement\"" w381 {
      tunnel: w387 -> [w396 w468 w634 w736 w749 w821]
      tunnel: w386 -> [w397 w467 w595 w737 w745 w817]
      tunnel: [w397 w433 w582 w729 w745 w817] -> w385
      tunnel: [w396 w441 w623 w730 w748 w820] -> w375
      tunnel: [w395 FALSE ("Global Stop") FALSE ("Global Stop") FALSE ("Global Stop") FALSE ("Global Stop") FALSE ("Global Stop")] -> w382
      tunnel: w380 -> [w395 _ _ _ _ _]
      tunnel: w379 -> [w394 w428 w615 w728 w747 w819]
      tunnel: [w394 w442 w624 w728 w747 w819] -> w378
      tunnel: w376 -> [_ w464 w631 _ _ _]
      frame #0 {
      }
      frame #1 {
        w411 = T18."Image File" ("Measurement Type")
        w440 = 32768 ("dimension size")
        # "TODO:\n- FIFO Read Flag Buffer Half Full?\n- Unselect in WS Tree on startup\n- end prog if error on startup"
        # "Image Intensity Array"
        n198 = control-ref of="Image"() -> (w406:refnum<vi>)
        n199 = Bundle("X-Position"="X-Position", "Y-Position"="Y-Position", "Z-Position"="Z-Position") -> (w402:T20)  [unwired: 1 in]
        n200 = Build Array("x-Pixel", "y-Pixel") -> (w400:u16[])
        n201 = Cluster To Array(cluster=w402) -> (array=w466:dbl[])
        n202 = call "PI_Scanner_In_Range.vi"("Picture size"="Picture size", "Picture size 2"="Picture size 2", "Upper Left"=w402, "Axis"="Axis") -> ("Picture size out"=w427:dbl, "Picture size out 2"=w426:dbl)  [unwired: 14 in]
        n203 = call "PI_MoveTo.vi"("System no."=w467, "Target position"=w466, "error in"=w468, "Move"=TRUE) -> ("System no. (dup)"=w450:i32, "error out"=w405:errorcluster)  [unwired: 13 in, 1 out]
        n204 = Build Array(w427, w426) -> (w401:dbl[])
        n205 = call "MTS_SetGraphScales.vi"("Pixels"=w400, "Axis"="Axis", "Picture Size"=w401, "error in (no error)"=w405, "Upper Left"=w402, "Image"=w406) -> ("error out"=w403:errorcluster)  [unwired: 5 in]
        n206 = call "MTS_GenFileComment.vi"("Measurement Type"=w411, "error in"=w428, "Upper Left"=w402, "Pixels"=w400, "Picture Size"=w401) -> ("error out"=w423:errorcluster, "Image Info"=w413:T21, "Comment"=w425:string)  [unwired: 4 in]
        n207 = control-ref of="WS File Tree"() -> (w412:refnum<vi>)
        n208 = call "PI_Image_Scanner_Prepare_Dlg.vi"("System no."=w450, "Picture Size"=w401, "Pixels"=w400, "Axis"="Axis", "Scanner Divider"="Scanner Divider", "error in"=w403, "Learning loop"="Learning loop") -> ("System no. (dup)"=w449:i32, "Measurement time [s]"=w445:i32, "error out"=w451:errorcluster)  [unwired: 6 in]
        n209 = local read "Workspace"() -> (w424:path)
        n210 = Index Array(array=w464) -> (element=w463:T22)  [unwired: 1 in]
        n211 = local write "Picture size"(w427) -> ()
        n212 = local write "Picture size 2"(w426) -> ()
        n213 = call "MTS_GetNextFileName.vi"("error in (no error)"=w423, "File Type"="pt3", "Measurement Type"="Image", "Workspace"=w424) -> ("error out"=w416:errorcluster, "Next File Name"=w415:path)  [unwired: 6 in]
        n214 = Unbundle By Name(w463) -> ("Dev"=w460:i32)
        n215 = call "PH_Set.vi"("Device List"=w464, "error in (no error)"=w451) -> ("pt3 header out"=w430:T23, "Count Rate"=w453:i32, "error out"=w432:errorcluster)  [unwired: 8 in, 3 out]
        n216 = Initialize Array(0 ("element"), "x-Pixel", "y-Pixel") -> (w454:i32[][])
        n217 = call "MTS_AddFileToWorkspace.vi"("File Name"=w415, "File Type"=T13."pt3 File", "Scan Axis"="Axis", "Measurement Type"=w411, "File Info"=w413, "error in (no error)"=w416, "Tree Refnum"=w412) -> ("File Name (dup)"=w399:path, "error out"=w414:errorcluster)  [unwired: 6 in, 1 out]
        n218 = call "MTS_CalcMeasTime.vi"("Scanner Divider"="Scanner Divider", "pt3 header in"=w430, "Measurement time [s]"=w445, "Count Rate"=w453) -> ("pt3 header out"=w429:T23, "Corrected Measurement time [s]"=→"Measure. time [s]":i32, "Calc Acq. Time (ms)"=w457:i32, "Overflow Interv. Time (s)"=w456:dbl, "Pixel Time (Laser Pulses)"=w452:i32)  [unwired: 7 in]
        n219 = call "PT3_Create.vi"("Save pt3"="Save Files", "error in"=w432, "Comment"=w425, "pt3 header in"=w429, "File Path"=w399) -> ("error out"=w431:errorcluster, "refnum out"=w420:refnum<file>)  [unwired: 5 in]
        n220 = call "PH_Start.vi"("Device Index"=w460, "Acq. Time"=w457, "error in (no error)"=w431) -> ("error out"=w461:errorcluster)  [unwired: 11 in, 1 out]
        n221 = To Unsigned Long Integer(number=w440) -> (unsigned 32bit integer=w437:u32)
        n222 = local write "Active pt3"(w399) -> ()
        n223 = Initialize Array(u32 0, w440) -> (w438:u32[])
        n224 = Unbundle By Name(w461) -> ("status"=w462:bool)
        n225 = Not(x=w462) -> (.not. x?=w459:bool)
        n226 = case shown="True" w459 {
          tunnel: [w522 w549] -> w443
          tunnel: [w524 w541] -> w434
          tunnel: w449 -> [w524 w538]
          tunnel: w461 -> [w523 w539]
          tunnel: w414 -> [w525 w547]
          tunnel: [w525 w546] -> w444
          tunnel: w460 -> [w521 w548]
          tunnel: w456 -> [_ w528]
          tunnel: w454 -> [_ w543]
          tunnel: w452 -> [_ w542]
          tunnel: "Axis" -> [_ w537]
          tunnel: w438 -> [_ w536]
          tunnel: w437 -> [_ w535]
          tunnel: [w520 w534] -> w436
          tunnel: [w520 w533] -> w435
          tunnel: w420 -> [w519 w532]
          tunnel: [w519 w531] -> w419
          tunnel: [0 ("Num Records Total") w530] -> w418
          tunnel: [0.0 w527] -> w417
          tunnel: [u64[] [] ("Histograms") w526] -> w410
          frame #0 {
            w520 = FALSE ("Stop Measurement")
            n227 = call "PH_Stop.vi"("Device Index"=w521, "error in (no error)"=w523) -> ("error out"=w522:errorcluster)  [unwired: 12 in, 1 out]
          }
          frame #1 {
            # "Overflow Interv. Time (s)"
            # "No Error"
            n228 = call "PI_Start_Wave_Gen.vi"("System no."=w538, "error in"=w539, "Axis"=w537) -> ("System no. (dup)"=w541:i32, "error out"=w540:errorcluster)  [unwired: 11 in]
            n229 = while {
              tunnel: w548 -> [w577]
              tunnel: w536 -> [w576]
              tunnel: w535 -> [w575]
              shift-right: [w561] -> w545
              shift-left: w540 -> [w578]
              shift-right: [w574] -> w546
              shift-left: w547 -> [w574]
              shift-right: [FALSE ("Reset")] -> _
              shift-left: TRUE ("Reset") -> [w570]
              tunnel: w543 -> [w567]
              tunnel: w542 -> [w563]
              tunnel: [w564] -> w534
              tunnel: [w554] -> w533
              tunnel: w532 -> [w558]
              tunnel: [w557] -> w531
              tunnel: [w556] -> w530
              tunnel: [w555] -> w529
              tunnel: [w550] -> w526
              stop <- w573 stop-if-true
              n230 = call "PH_FIFORead.vi"("Device Index"=w577, "Buffer In"=w576, "Count"=w575, "error in (no error)"=w578) -> ("OK"=w565:bool, "Buffer Out"=w559:u32[], "Data Count"=w560:i32, "FiFo Overrun"=w564:bool, "error out"=w562:errorcluster)  [unwired: 7 in]
              n231 = Wait (ms)(milliseconds to wait=u32 10) -> ()  [unwired: 1 out]
              n232 = local write "FiFo Overrun"(w564) -> ()
              n233 = local read "Global Stop"() -> (w552:bool)
              n234 = Unbundle(w562) -> ("status"=w572:bool)  [unwired: 2 out]
              n235 = call "PH_ToImage.vi"("Data In"=w559, "Reset"=w570, "Image Array In"=w567, "Data Count"=w560, "Pixel Time (Laser Pulses)"=w563) -> ("Image Array Out"=→"Image":i32[][], "Histograms"=→"Histogram":i32[][], "Total Photon Count"=w550:u64[], "Total Oveflow Count"=w555:u64, "Num Records Total"=w556:i32, "Traces"=→"Trace":i32[][])  [unwired: 4 in, 1 out]
              n236 = call "PT3_Write.vi"("error in"=w562, "Data Count"=w560, "Data in"=w559, "refnum in"=w558) -> ("error out"=w561:errorcluster, "refnum out"=w557:refnum<file>)  [unwired: 6 in]
              n237 = local read "Stop Measurement"() -> (w553:bool)
              n238 = Compound Arithmetic op=OR(invert w565, w572, w552, w553) -> (w573:bool)
              n239 = Or(x=w553, y=w552) -> (x .or. y?=w554:bool)
            }
            n240 = Multiply(x=w528, y=w529) -> (x*y=w527:dbl)
            n241 = call "PH_Stop.vi"("Device Index"=w548, "error in (no error)"=w545) -> ("error out"=w549:errorcluster)  [unwired: 12 in, 1 out]
          }
        }
        n242 = control-ref of="WS File Tree"() -> (w408:refnum<vi>)
        n243 = flat-sequence {
          tunnel: w444 -> [w504]
          tunnel: w443 -> [w500]
          tunnel: [w504] -> w442
          tunnel: [w478] -> w441
          tunnel: w436 -> [w502]
          tunnel: w435 -> [w489]
          tunnel: w434 -> [w499]
          tunnel: [w498] -> w433
          tunnel: w419 -> [w495]
          tunnel: w418 -> [w494]
          tunnel: w417 -> [w487]
          tunnel: w410 -> [w488]
          tunnel: "Save Files" -> [w477]
          tunnel: w399 -> [w476]
          tunnel: w408 -> [w475]
          frame #0 {
            # "Count Rate (per s)"
            # "Stop WaveGen\nif Aborted"
            # "Finish after Aquire Image"
            n244 = Or(x=w489, y=w502) -> (x .or. y?=w501:bool)
            n245 = case shown="False" w501 {
              tunnel: w500 -> [w507 w515]
              tunnel: w499 -> [w506 w514]
              tunnel: [w506 w513] -> w498
              tunnel: [w507 w512] -> w496
              tunnel: [enum16{"timeover", "manual", "overflow"}."timeover" ("Stop Reason") w510] -> w490
              tunnel: w489 -> [_ w508]
              frame #0 {
              }
              frame #1 {
                n246 = call "PI_Stop_Wave_Gen.vi"("System no."=w514, "error in"=w515) -> ("System no. (dup)"=w513:i32, "error out"=w512:errorcluster)  [unwired: 12 in]
                n247 = Select(t=enum16{"timeover", "manual", "overflow"}."manual" ("Stop Reason"), s=w508, f=enum16{"timeover", "manual", "overflow"}."overflow" ("Stop Reason")) -> (s? t:f=w510:enum16{"timeover", "manual", "overflow"})
              }
            }
            n248 = Multiply(x=w487, y=1000.0) -> (x*y=w492:dbl)
            n249 = Divide(x=w488, y=w487) -> (x/y=w486:dbl[])
            n250 = To Long Integer(number=w492) -> (32bit integer=w491:i32)
            n251 = To Long Integer(number=w486) -> (32bit integer=w485:i32[])
            n252 = property on="Aquire Image" class="Bool"("BoolText.Text"="Aquire Image" ("Caption.Text"), "BoolText.TextColor"=u32 0 ("Boolean Text.Colors:FG Color")) -> ()  [unwired: 2 in, 2 out]
            n253 = Index Array(array=w485, index #1=0 ("index"), index #2=1 ("index")) -> (element #1=w482:i32, element #2=w481:i32)
            n254 = local read "Image"() -> (w480:i32[][])
            n255 = call "PT3_Finish.vi"("Input 1 Rate"=w481, "Input 0 Rate"=w482, "Stop Reason"=w490, "error in"=w496, "Num Records"=w494, "Stop After (ms)"=w491, "refnum in"=w495) -> ("error out"=w479:errorcluster)  [unwired: 4 in]
            n256 = call "MTS_SaveImagePng.vi"("Save .png"=w477, "Tree Refnum"=w475, ".pt3 File Name"=w476, "error in"=w479, "Image"=w480) -> ("error out"=w478:errorcluster)  [unwired: 6 in]
          }
        }
      }
      frame #2 {
        w588 = T18."Point Measurement" ("Measurement Type")
        w622 = 32768 ("dimension size")
        n257 = local read "X-Position"() -> (w598:dbl)
        n258 = local read "Z-Position"() -> (w597:dbl)
        n259 = local read "Y-Position"() -> (w596:dbl)
        n260 = local read "Workspace"() -> (w613:path)
        n261 = control-ref of="WS File Tree"() -> (w600:refnum<vi>)
        n262 = Index Array(array=w631) -> (element=w630:T22)  [unwired: 1 in]
        n263 = Bundle("X-Position"=w598, "Z-Position"=w597, "Y-Position"=w596) -> (w580:T24)  [unwired: 1 in]
        n264 = Cluster To Array(cluster=w580) -> (array=w633:dbl[])
        n265 = Unbundle By Name(w630) -> ("Dev"=w583:i32)
        n266 = call "PI_MoveTo.vi"("System no."=w595, "Target position"=w633, "error in"=w634, "Move"=TRUE) -> ("System no. (dup)"=w582:i32, "error out"=w599:errorcluster)  [unwired: 13 in, 1 out]
        n267 = call "MTS_GenFileComment.vi"("Measurement Type"=w588, "error in"=w615, "Upper Left"=w580) -> ("error out"=w612:errorcluster, "Image Info"=w601:T21, "Comment"=w614:string)  [unwired: 6 in]
        n268 = call "PH_Set.vi"("Device List"=w631, "error in (no error)"=w599) -> ("pt3 header out"=w591:T23, "Count Rate"=w592:i32, "error out"=w585:errorcluster)  [unwired: 8 in, 3 out]
        n269 = Bundle By Name(cluster=w591, "AcquisitionTime (ms)"="Measurement Time (ms)") -> (w590:T23)
        n270 = Reciprocal(x=w592) -> (1/x=w594:dbl)
        n271 = call "MTS_GetNextFileName.vi"("error in (no error)"=w612, "File Type"="pt3", "Measurement Type"="Point", "Workspace"=w613) -> ("error out"=w605:errorcluster, "Next File Name"=w604:path)  [unwired: 6 in]
        n272 = Scale By Power Of 2(n=16, x=w594) -> (x*2^n=w581:dbl)
        n273 = case shown="True" FALSE {
          tunnel: w585 -> [w636 w643]
          tunnel: [w636 w642] -> w584
          tunnel: w583 -> [_ w641]
          tunnel: w582 -> [_ w640]
          tunnel: w581 -> [_ w639]
          tunnel: w580 -> [_ w638]
          frame #0 {
          }
          frame #1 {
            # "Auto Z"
            n274 = call "MTS_AutoZPos.vi"("PH Dev"=w641, "OFlow Interv [s]"=w639, "PI System no."=w640, "error in"=w643, "Start Point"=w638) -> ("New Z"=w637:dbl, "error out"=w642:errorcluster)  [unwired: 8 in, 1 out]
            n275 = local write "Z-Position"(w637) -> ()
          }
        }
        n276 = call "MTS_AddFileToWorkspace.vi"("File Name"=w604, "File Type"=T13."pt3 File", "Measurement Type"=w588, "File Info"=w601, "error in (no error)"=w605, "Tree Refnum"=w600) -> ("File Name (dup)"=w602:path, "error out"=w603:errorcluster)  [unwired: 7 in, 1 out]
        n277 = call "PT3_Create.vi"("error in"=w584, "Comment"=w614, "pt3 header in"=w590, "File Path"=w602) -> ("error out"=w616:errorcluster, "refnum out"=w609:refnum<file>)  [unwired: 6 in]
        n278 = call "PH_Start.vi"("Device Index"=w583, "Acq. Time"="Measurement Time (ms)", "error in (no error)"=w616) -> ("error out"=w628:errorcluster)  [unwired: 11 in, 1 out]
        n279 = To Unsigned Long Integer(number=w622) -> (unsigned 32bit integer=w619:u32)
        n280 = Initialize Array(u32 0, w622) -> (w620:u32[])
        n281 = Unbundle By Name(w628) -> ("status"=w629:bool)
        n282 = Not(x=w629) -> (.not. x?=w627:bool)
        n283 = case shown="True" w627 {
          tunnel: [w680 w700] -> w625
          tunnel: w628 -> [w681 w684]
          tunnel: w603 -> [w682 w698]
          tunnel: [w682 w697] -> w626
          tunnel: w583 -> [w679 w699]
          tunnel: w581 -> [_ w686]
          tunnel: w620 -> [_ w694]
          tunnel: w619 -> [_ w693]
          tunnel: [w678 w692] -> w618
          tunnel: [w678 w691] -> w617
          tunnel: w609 -> [w677 w690]
          tunnel: [w677 w689] -> w608
          tunnel: [0 ("Num Records Total") w688] -> w607
          tunnel: [0.0 w685] -> w606
          tunnel: [u64[] [] ("Total Photon Count") w683] -> w587
          frame #0 {
            w678 = FALSE ("Stop Measurement")
            n284 = call "PH_Stop.vi"("Device Index"=w679, "error in (no error)"=w681) -> ("error out"=w680:errorcluster)  [unwired: 12 in, 1 out]
          }
          frame #1 {
            # "Overflow Interv. Time (s)"
            # "No Error"
            n285 = while {
              tunnel: w699 -> [w725]
              tunnel: w694 -> [w724]
              tunnel: w693 -> [w723]
              shift-right: [w713] -> w696
              shift-left: w684 -> [w726]
              shift-right: [w722] -> w697
              shift-left: w698 -> [w722]
              shift-right: [FALSE ("Reset")] -> _
              shift-left: TRUE ("Reset") -> [w718]
              tunnel: [w715] -> w692
              tunnel: [w706] -> w691
              tunnel: w690 -> [w710]
              tunnel: [w709] -> w689
              tunnel: [w708] -> w688
              tunnel: [w707] -> w687
              tunnel: [w701] -> w683
              stop <- w721 stop-if-true
              n286 = call "PH_FIFORead.vi"("Device Index"=w725, "Buffer In"=w724, "Count"=w723, "error in (no error)"=w726) -> ("OK"=w716:bool, "Buffer Out"=w711:u32[], "Data Count"=w712:i32, "FiFo Overrun"=w715:bool, "error out"=w714:errorcluster)  [unwired: 7 in]
              n287 = Wait (ms)(milliseconds to wait=u32 10) -> ()  [unwired: 1 out]
              n288 = local write "FiFo Overrun"(w715) -> ()
              n289 = local read "Global Stop"() -> (w704:bool)
              n290 = Unbundle(w714) -> ("status"=w720:bool)  [unwired: 2 out]
              n291 = call "PH_ToImage.vi"("Data In"=w711, "Reset"=w718, "Data Count"=w712) -> ("Histograms"=w703:i32[][], "Total Photon Count"=w701:u64[], "Total Oveflow Count"=w707:u64, "Num Records Total"=w708:i32, "Traces"=w702:i32[][])  [unwired: 6 in, 2 out]
              n292 = call "PT3_Write.vi"("error in"=w714, "Data Count"=w712, "Data in"=w711, "refnum in"=w710) -> ("error out"=w713:errorcluster, "refnum out"=w709:refnum<file>)  [unwired: 6 in]
              n293 = local read "Stop Measurement"() -> (w705:bool)
              n294 = local write "Histogram"(w703) -> ()
              n295 = local write "Trace"(w702) -> ()
              n296 = Compound Arithmetic op=OR(invert w716, w720, w704, w705) -> (w721:bool)
              n297 = Or(x=w705, y=w704) -> (x .or. y?=w706:bool)
            }
            n298 = Multiply(x=w686, y=w687) -> (x*y=w685:dbl)
            n299 = call "PH_Stop.vi"("Device Index"=w699, "error in (no error)"=w696) -> ("error out"=w700:errorcluster)  [unwired: 12 in, 1 out]
          }
        }
        n300 = flat-sequence {
          tunnel: w626 -> [w666]
          tunnel: w625 -> [w662]
          tunnel: [w666] -> w624
          tunnel: [w659] -> w623
          tunnel: w618 -> [w664]
          tunnel: w617 -> [w652]
          tunnel: w608 -> [w658]
          tunnel: w607 -> [w657]
          tunnel: w606 -> [w647]
          tunnel: w587 -> [w646]
          frame #0 {
            # "Finish after Measurement"
            n301 = Or(x=w652, y=w664) -> (x .or. y?=w663:bool)
            n302 = case shown="True" w663 {
              tunnel: w662 -> [w668 w669]
              tunnel: [w668 w669] -> w660
              tunnel: [enum16{"timeover", "manual", "overflow"}."timeover" ("Stop Reason") w672] -> w653
              tunnel: w652 -> [_ w670]
              frame #0 {
              }
              frame #1 {
                n303 = Select(t=enum16{"timeover", "manual", "overflow"}."manual" ("Stop Reason"), s=w670, f=enum16{"timeover", "manual", "overflow"}."overflow" ("Stop Reason")) -> (s? t:f=w672:enum16{"timeover", "manual", "overflow"})
              }
            }
            n304 = Multiply(x=w647, y=1000.0) -> (x*y=w655:dbl)
            n305 = Divide(x=w646, y=w647) -> (x/y=w648:dbl[])
            n306 = To Long Integer(number=w655) -> (32bit integer=w654:i32)
            n307 = To Long Integer(number=w648) -> (32bit integer=w649:i32[])
            n308 = property on="Point Measurement" class="Bool"("BoolText.Text"="Point Measurement" ("Caption.Text"), "BoolText.TextColor"=u32 0 ("Boolean Text.Colors:FG Color")) -> ()  [unwired: 2 in, 2 out]
            n309 = Index Array(array=w649, index #1=0 ("index"), index #2=1 ("index")) -> (element #1=w645:i32, element #2=w644:i32)
            n310 = call "PT3_Finish.vi"("Input 1 Rate"=w644, "Input 0 Rate"=w645, "Stop Reason"=w653, "error in"=w660, "Num Records"=w657, "Stop After (ms)"=w654, "refnum in"=w658) -> ("error out"=w659:errorcluster)  [unwired: 4 in]
          }
        }
      }
      frame #3 {
        n311 = local read "X-Position"() -> (w735:dbl)
        n312 = local read "Y-Position"() -> (w734:dbl)
        n313 = local read "Z-Position"() -> (w733:dbl)
        n314 = Build Array(w735, w734, w733) -> (w732:dbl[])
        n315 = call "PI_MoveTo.vi"("System no."=w737, "Target position"=w732, "error in"=w736, "Move"=TRUE) -> ("System no. (dup)"=w729:i32, "error out"=w730:errorcluster)  [unwired: 13 in, 1 out]
      }
      frame #4 {
        n316 = local read "Active pt3"() -> (w743:path)
        n317 = call "MTS_GetFileFromWS.vi"(".pt3 File Name"=w743) -> ("File Header"=w742:T17)  [unwired: 9 in, 1 out]
        n318 = Unbundle By Name(w742) -> ("Measurement Type"=w741:T18, "Pixels"=w738:i32[])
        n319 = Equal?(x=T18."Image File" ("Measurement Type"), y=w741) -> (x = y?=w739:bool)
        n320 = control-ref of="WS File Tree"() -> (w744:refnum<vi>)
        n321 = case shown="True" w739 {
          tunnel: w749 -> [w750 w779]
          tunnel: w743 -> [_ w778]
          tunnel: w743 -> [_ w761]
          tunnel: [w750 w751] -> w748
          tunnel: w744 -> [_ w758]
          tunnel: w738 -> [_ w757]
          frame #0 {
          }
          frame #1 {
            # "Image Intensity Array"
            # "Image Intensity Array"
            n322 = call "PT3_Open.vi"("error in"=w779, "File Path"=w778) -> ("error out"=w771:errorcluster, "Header"=w775:T25, "refnum out"=w777:refnum<file>)  [unwired: 4 in, 3 out]
            n323 = Index Array(array=w757, index #2=1 ("index")) -> (element #1=w754:i32, element #2=w755:i32)  [unwired: 1 in]
            n324 = Unbundle By Name(w775) -> ()  [unwired: 15 out]
            n325 = Initialize Array(0 ("element"), w754, w755) -> (w773:i32[][])
            n326 = while {
              tunnel: w777 -> [w805]
              shift-right: [FALSE ("Start From Top")] -> _
              shift-left: TRUE ("Start From Top") -> [w799]
              shift-right: [w798] -> w770
              shift-left: w771 -> [w793]
              tunnel: [w797] -> w769
              tunnel: w773 -> [w796]
              tunnel: [w795] -> w772
              tunnel: [w794] -> _
              stop <- w802 stop-if-true
              n327 = call "PT3_Read.vi"("Start From Top"=w799, "error in"=w793, "Data count"=10000, "refnum in"=w805) -> ("error out"=w798:errorcluster, "Data out"=w801:u32[], "refnum out"=w797:refnum<file>, "EOF?"=w802:bool)  [unwired: 4 in]
              n328 = Array Size(array=w801) -> (size(s)=w800:i32)
              n329 = call "MTS_ToImageOffline.vi"("Data In"=w801, "Reset"=w799, "Image Array In"=w796, "Data Count"=w800) -> ("Image Array Out"=w794:i32[][], "Histograms"=w795:i32[][])  [unwired: 2 in, 8 out]
            }
            n330 = call "MTS_SelectTCSPCBinning.vi"("Histograms in"=w772) -> ("TCSPC Binning"=w765:i32[][], "Colors"=w759:u32[], "Active"=w760:bool[])  [unwired: 1 in, 7 out]
            n331 = Initialize Array(0 ("element"), 4 ("dimension size"), w754, w755) -> (w766:i32[][][])
            n332 = while {
              tunnel: w769 -> [w792]
              shift-right: [FALSE ("Start From Top")] -> _
              shift-left: TRUE ("Start From Top") -> [w786]
              shift-right: [w785] -> w763
              shift-left: w770 -> [w781]
              tunnel: [w784] -> w752
              tunnel: w766 -> [w783]
              tunnel: [w782] -> w762
              tunnel: w765 -> [w780]
              stop <- w789 stop-if-true
              n333 = call "PT3_Read.vi"("Start From Top"=w786, "error in"=w781, "Data count"=10000, "refnum in"=w792) -> ("error out"=w785:errorcluster, "Data out"=w788:u32[], "refnum out"=w784:refnum<file>, "EOF?"=w789:bool)  [unwired: 4 out]
              n334 = Array Size(array=w788) -> (size(s)=w787:i32)
              n335 = call "MTS_ToColorImage.vi"("Data In"=w788, "Reset"=w786, "Image Array In"=w783, "Data Count"=w787, "TCSPC Binning"=w780) -> ("Image Array Out"=w782:i32[][][])  [unwired: 2 in, 8 out]
            }
            n336 = call "MTS_SaveColorImagePng.vi"("Tree Refnum"=w758, ".pt3 File Name"=w761, "error in"=w763, "Colors"=w759, "Active"=w760, "Image"=w762) -> ("error out"=w753:errorcluster)  [unwired: 5 in]
            n337 = Close File(refnum=w752, error in=w753) -> (error out=w751:errorcluster)  [unwired: 1 out]
          }
        }
      }
      frame #5 {
        n338 = local read "Active pt3"() -> (w816:path)
        n339 = call "MTS_GetFileFromWS.vi"(".pt3 File Name"=w816) -> ("File Header"=w815:T17)  [unwired: 9 in, 1 out]
        n340 = Unbundle By Name(w815) -> ("Measurement Type"=w814:T18, "Pixels"=w811:i32[], "Picture Size"=w810:dbl[], "Upper Left"=w809:T19, "Scan Axis"=w808:enum32{"x-y", "x-z", "y-z"})
        n341 = call "MTS_ScannerXYZToImageXY.vi"("Axis"=w808, "Scanner XYZ"=w809) -> ("Image Y"=w806:dbl, "Image X"=w807:dbl)
        n342 = Equal?(x=T18."Image File" ("Measurement Type"), y=w814) -> (x = y?=w812:bool)
        n343 = case shown="True" w812 {
          tunnel: w821 -> [w822 w839]
          tunnel: w816 -> [_ _]
          tunnel: w816 -> [_ _]
          tunnel: [w822 w838] -> w820
          tunnel: w811 -> [_ w846]
          tunnel: w810 -> [_ w845]
          tunnel: w807 -> [_ w829]
          tunnel: w806 -> [_ w832]
          frame #0 {
          }
          frame #1 {
            w841 = 0.6  # psf width [um]
            w844 = 1 ("index")
            # "Gauss Width"
            # "Pixel Size [um]"
            n344 = Index Array(array=w846, index #2=w844) -> (element #1=w842:i32, element #2=w835:i32)  [unwired: 1 in]
            n345 = Index Array(array=w845, index #2=w844) -> (element #1=w843:dbl, element #2=w834:dbl)  [unwired: 1 in]
            n346 = local read "Image"() -> (w837:i32[][])
            n347 = Divide(x=w843, y=w842) -> (x/y=w824:dbl)
            n348 = Divide(x=w834, y=w835) -> (x/y=w833:dbl)
            n349 = Reciprocal(x=w824) -> (1/x=w823:dbl)
            n350 = To Double Precision Float(number=w837) -> (double precision float=w836:dbl[][])
            n351 = Multiply(x=w823, y=w841) -> (x*y=w840:dbl)
            n352 = script code="mask = GenGauss2D(gw);\n[err, bim, cim, sim, yc, xc, bc, cc, sc, len, imm] = FindPatternCP(Image, mask, [], [], [], 1.5);"("??"=w839, "gw"=w840, "Image"=w836) -> ("??"=w838:errorcluster, "xc"=w830:dbl[], "yc"=w831:dbl[])
            n353 = Multiply(x=w824, y=w830) -> (x*y=w828:dbl[])
            n354 = Multiply(x=w831, y=w833) -> (x*y=w827:dbl[])
            n355 = Add(x=w829, y=w828) -> (x+y=→"Pattern X":dbl[])
            n356 = Add(x=w827, y=w832) -> (x+y=→"Pattern Y":dbl[])
          }
        }
      }
    }
    n357 = Unbundle(w375) -> ("status"=w374:bool)  [unwired: 2 out]
    n358 = flat-sequence {
      tunnel: w378 -> [w393]
      tunnel: [w393] -> w377
      frame #0 {
        n359 = control-ref of="ShowTab"() -> (w390:refnum<vi>)
        n360 = local write "Do Measurement"(T11."No Measurement" ("Do Measurement")) -> ()
        n361 = local write "MeasRunig"(FALSE ("Measurement Running")) -> ()
        n362 = call "MTS_ShowHideTabs.vi"("Action"=enum16{"Show All", "Hide Tab", "Show Tab"}."Show All", "ShowTab"=w390) -> ()  [unwired: 8 in, 2 out]
      }
    }
    n363 = local read "Global Stop"() -> (w384:bool)
    n364 = Compound Arithmetic op=OR(w374, w382, w384) -> (w383:bool)
  }
  n365 = while {
    tunnel: w18 -> [w857]
    shift-right: [w856] -> _
    shift-left: w17 -> [w858]
    stop <- w855 stop-if-true
    n366 = Wait (ms)(milliseconds to wait=u32 50) -> ()  [unwired: 1 out]
    n367 = case shown="True" "SCANNER EMERGENCY" {
      tunnel: w857 -> [_ w863]
      tunnel: w858 -> [w861 w864]
      tunnel: [w861 w865] -> w856
      frame #0 {
        n368 = Wait Until Next ms Multiple(millisecond multiple=u32 100) -> ()  [unwired: 1 out]
      }
      frame #1 {
        n369 = call "PI_Stop_Wave_Gen.vi"("System no."=w863, "error in"=w864) -> ("error out"=w862:errorcluster)  [unwired: 12 in, 1 out]
        n370 = flat-sequence {
          tunnel: [w866] -> w865
          tunnel: w862 -> [w866]
          frame #0 {
            n371 = One Button Dialog(message="Emergency scanner stop appeared!!!\nCheck scanner settings before continue!!!") -> ()  [unwired: 2 out]
          }
        }
      }
    }
    n372 = local read "Global Stop"() -> (w855:bool)
  }
  n373 = call "DT3120_CloseDevice.vi"("error in (no error)"=w11, "lpDevId"=w9) -> ("error out"=w4:errorcluster)  [unwired: 9 out]
  n374 = call "IMAQ Dispose"("Image"=w3, "error in (no error)"=w4) -> ("error out"=w2:errorcluster)  [unwired: 4 in]
  n375 = flat-sequence {
    tunnel: w2 -> [w870]
    tunnel: [w868] -> w1
    frame #0 {
      n376 = call "CAN USB Close.vi"() -> ("Error Number"=w869:u32)  [unwired: 1 in]
      n377 = call <vilib>:"Error Cluster From Error Code.vi"("error in (no error)"=w870, "error message (\"\")"="PCAN Close Error" ("error message (\"\")"), "error code (0)"=w869) -> ("error out"=w868:errorcluster)  [unwired: 6 in]
    }
  }
  n378 = call <vilib>:"Merge Errors.vi"("error in 2 (no error)"=w8, "error in 1 (no error)"=w1) -> ("error out"=w7:errorcluster)  [unwired: 5 in]
  n379 = flat-sequence {
    tunnel: w14 -> [w872]
    tunnel: [w872] -> w13
    frame #0 {
      n380 = local write "Global Stop"(TRUE ("Global Stop")) -> ()
    }
  }
  n381 = call "Close connection if open.vi"("System no."=w23, "error in"=w13) -> ("error out"=w22:errorcluster)  [unwired: 16 in, 1 out]
  n382 = call <vilib>:"Merge Errors.vi"("error in 3 (no error)"=w22, "error in 2 (no error)"=w19, "error in 1 (no error)"=w7) -> ("error out"=w21:errorcluster)  [unwired: 4 in]
  n383 = call <vilib>:"Simple Error Handler.vi"("error in (no error)"=w21) -> ()  [unwired: 4 in, 5 out]
